vi "Set Axis Properties.vi"(8 "error in":errorcluster, 10 "Prop String":string, 11 "address":string="192.168.0.90") -> (0 "error out":errorcluster)   [LabVIEW 2017]
panel:
  out "For Documentation Only":string="Content-type: text/plain\n\nroot.ImageSource.I0.Sensor.WhiteBalance=auto\nroot.ImageSource.I0.Sensor.Exposure=auto\nroot.ImageSource.I0.Sensor.ExposurePriority=50\nroot.ImageSource.I0.Sensor.Brightness=60\nroot.ImageSource.I0.Sensor.ColorLevel=50\nroot.ImageSource.I0.Sensor.Sharpness=0\nroot.ImageSource.I0.Sensor.BlacklevelCorrection=0\n"
  out "Camera Request":string
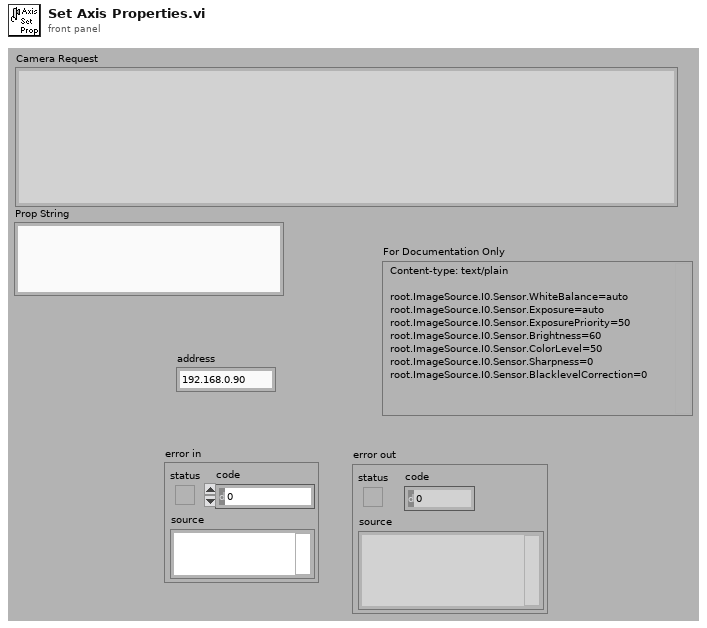
[diagram p1: front panel]
types:
  T1 = enum16{"Standard", "Buffered", "CRLF", "Immediate"}
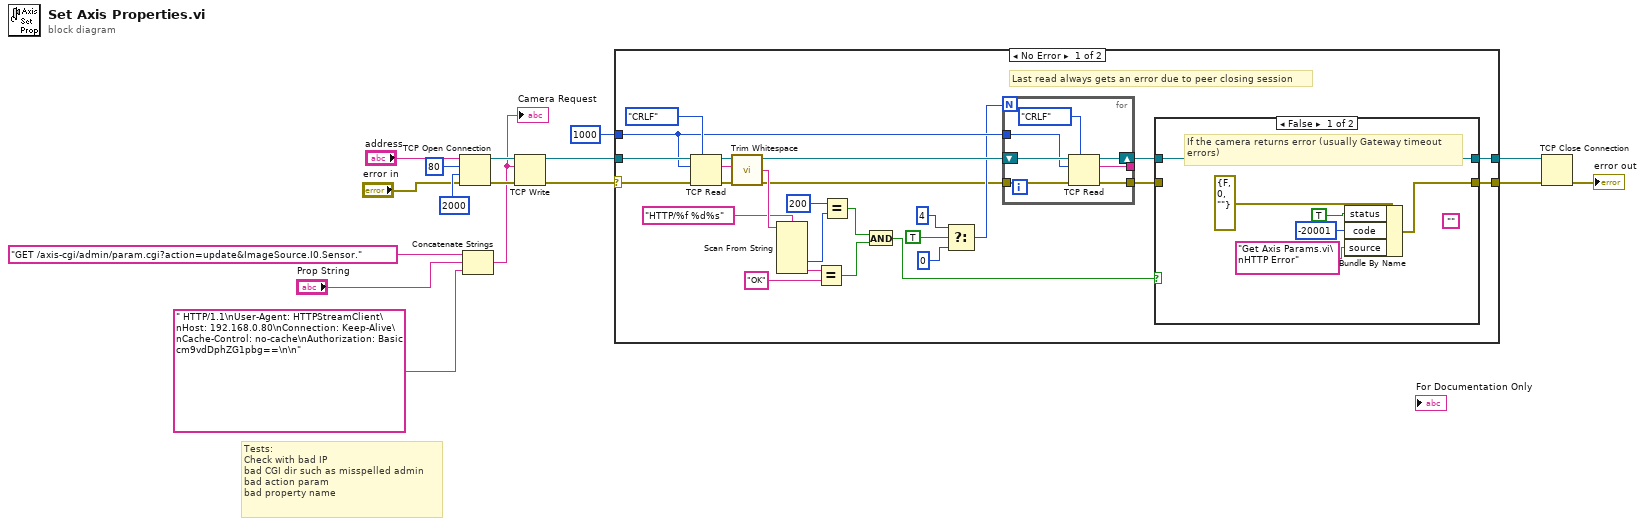
[diagram p0: block diagram]
diagram:
  # "Tests:\nCheck with bad IP\nbad CGI dir such as misspelled admin\nbad action param\nbad property name"
  n1 = TCP Open Connection(address="address", remote port or service name=u16 80, timeout ms (60000)=2000, error in (no error)="error in") -> (connection ID=w11:refnum<k5>, error out=w6:errorcluster)  [unwired: 1 in]
  n2 = Concatenate Strings("GET /axis-cgi/admin/param.cgi?action=update&ImageSource.I0.Sensor.", "Prop String", " HTTP/1.1\nUser-Agent: HTTPStreamClient\nHost: 192.168.0.80\nConnection: Keep-Alive\nCache-Control: no-cache\nAuthorization: Basic cm9vdDphZG1pbg==\n\n") -> (w1:string)
  "Camera Request" <- w1
  n3 = TCP Write(connection ID=w11, data in=w1, error in (no error)=w6) -> (connection ID out=w9:refnum<k5>, error out=w10:errorcluster)  [unwired: 1 in, 1 out]
  n4 = case shown="No Error" w10 {
    selector: w10 -> [w21 w56]
    tunnel: [w40 w56] -> w8
    tunnel: w9 -> [w37 w55]
    tunnel: 1000 ("bytes to read") -> [w26 _]
    tunnel: [w39 w55] -> w4
    frame No Error {
      # "Last read always gets an error due to peer closing session"
      n5 = TCP Read(connection ID=w37, bytes to read=w26, error in (no error)=w21, 7:T1."CRLF" ("mode (standard)")) -> (connection ID out=w27:refnum<k5>, data out=w38:string, error out=w20:errorcluster)  [unwired: 1 in]
      n6 = call <vilib>:"Trim Whitespace.vi"("string"=w38) -> ("trimmed string"=w35:string)  [unwired: 1 in]
      n7 = Scan From String(format string="HTTP/%f %d%s", input string=w35) -> (output 2=w33:i32, output 3=w31:string)  [unwired: 6 in, 3 out]
      n8 = Equal?(x=w31, y="OK" ("format string")) -> (x = y?=w29:bool)
      n9 = Equal?(x=200, y=w33) -> (x = y?=w28:bool)
      n10 = And(x=w28, y=w29) -> (x .and. y?=w18:bool)
      n11 = Select(t=4, s=TRUE, f=0) -> (s? t:f=w23:i32)
      n12 = for {
        N: w23 -> [_]
        tunnel: w26 -> [w45]
        shift-right: [w44] -> w22
        shift-left: w27 -> [w46]
        tunnel: w20 -> [w43]
        tunnel: [w42] -> w19
        tunnel: [w41] -> _
        n13 = TCP Read(connection ID=w46, bytes to read=w45, error in (no error)=w43, 7:T1."CRLF" ("mode (standard)")) -> (connection ID out=w44:refnum<k5>, data out=w41:string, error out=w42:errorcluster)  [unwired: 1 in]
      }
      n14 = case shown="False" w18 {
        tunnel: w22 -> [w48 w54]
        tunnel: w19 -> [_ _]
        tunnel: [w53 _] -> w40
        tunnel: [w48 w54] -> w39
        frame False {
          (unwired) ""
          # "If the camera returns error (usually Gateway timeout\nerrors)"
          n15 = Bundle By Name(cluster=errorcluster {"status"=FALSE, "code"=0, "source"=""} ("error in"), "status"=TRUE, "code"=-20001, "source"="Get Axis Params.vi\nHTTP Error") -> (w53:errorcluster)
        }
        frame True {
        }
      }
    }
    frame Error {
    }
  }
  n16 = TCP Close Connection(connection ID=w4, error in (no error)=w8) -> (error out=→"error out":errorcluster)  [unwired: 1 in, 1 out]
